vi "1.vi"() -> ()   [LabVIEW 2019]
uses:
  <vilib>/imath/engines/lvmath/Plug In/_Char/NIMS_CH_character datatype.ctl
  <vilib>/imath/engines/lvmath2/RunTimeEngine/Managers/WorkSpace/UID Generator.vi
  <vilib>/imath/engines/lvmath2/RunTimeEngine/BuiltInFunctions/close/NIMS_close(Enums).vi
  <vilib>/imath/engines/lvmath2/RunTimeEngine/RangeToken/NIMS_Range.vi
  <instcachedir>/0/NIMS_Range_FADF6ADDA3E145BB934C8BD4C7DAAB97.lvgen/NIMS_Range_FADF6ADDA3E145BB934C8BD4C7DAAB97_000.vi
  <vilib>/imathl/engines/lvmath/Functions/Error Handling/Create Error.vi
  <vilib>/imath/engines/lvmath/Plug In/_Char/NIMS_CH_Character RV to String.vi
  <vilib>/imath/engines/lvmath2/RunTimeEngine/BuiltInFunctions/random/NIMS_random.vi
  <vilib>/imath/engines/lvmath2/RunTimeEngine/IndexRead/NIMS M(S).vi
  <instcachedir>/0/NIMS M(S)_B826C018497E4940AE96BD27B540B6FB.lvgen/NIMS M(S)_B826C018497E4940AE96BD27B540B6FB_000.vi
  <vilib>/imath/engines/lvmath2/RunTimeEngine/ArithmeticOperatorToken/NIMS_ArithmeticOperator_plus.vi
  <instcachedir>/0/NIMS_ArithmeticOperator_plus_5C9385B0197D46E2B844C41E02F9EC39.lvgen/NIMS_ArithmeticOperator_plus_5C9385B0197D46E2B844C41E02F9EC39_004.vi
  <vilib>/imath/engines/lvmath2/RunTimeEngine/ErrorHandling/NIMS_Create Error From Enums.vi
  <vilib>/imath/engines/lvmath2/RunTimeEngine/BuiltInFunctions/randnormal/NIMS_randnormal(1,I32).vi
  <vilib>/imath/engines/lvmath2/RunTimeEngine/ErrorHandling/NIMS_Error From Error Code.vi
  <vilib>/imath/engines/lvmath/Functions/Error Handling/MergeErrorsWrapper.vi
  <vilib>/imath/engines/lvmath2/RunTimeEngine/BuiltInFunctions/fft/NIMS_fft(GV).vi
  <instcachedir>/0/NIMS_fft(GV)_4C6467FC22F84E4BA42517A07EF978B0.lvgen/NIMS_fft(GV)_4C6467FC22F84E4BA42517A07EF978B0_000.vi
  <vilib>/imath/engines/lvmath2/RunTimeEngine/BuiltInFunctions/abs/NIMS_abs(signed).vi
  <instcachedir>/0/NIMS_abs(signed)_C4FCB8E6058B49B797C7C8D53CA5F6EC.lvgen/NIMS_abs(signed)_C4FCB8E6058B49B797C7C8D53CA5F6EC_006.vi
  <vilib>/imath/engines/lvmath2/RunTimeSupport/NIMS_Error if Not Equal.vi
  <vilib>/imath/engines/lvmath2/RunTimeEngine/IndexRead/NIMS V(V).vi
  <instcachedir>/0/NIMS V(V)_298D9CB7BFEB42B8BC8D9C3C28AE8C70.lvgen/NIMS V(V)_298D9CB7BFEB42B8BC8D9C3C28AE8C70_000.vi
  <vilib>/imath/engines/lvmath2/RunTimeEngine/BuiltInFunctions/psd_periodogram/NIMS_psd_periodogram().vi
  <instcachedir>/0/NIMS_psd_periodogram()_F7AFC2F0C6104ABD8A95B4677FDE116B.lvgen/NIMS_psd_periodogram()_F7AFC2F0C6104ABD8A95B4677FDE116B_000.vi
  <vilib>/imath/engines/lvmath2/RunTimeEngine/Managers/SymbolTable/Clear UID.vi
  <vilib>/imath/engines/lvmath2/RunTimeEngine/NodeEndStatement/NIMS_NodeEndStatement_Output.vi
  <instcachedir>/0/NIMS_NodeEndStatement_Output_53EC0D466D134D7ABD903AC30B43404B.lvgen/NIMS_NodeEndStatement_Output_53EC0D466D134D7ABD903AC30B43404B_005.vi
  <instcachedir>/0/NIMS_NodeEndStatement_Output_53EC0D466D134D7ABD903AC30B43404B.lvgen/NIMS_NodeEndStatement_Output_53EC0D466D134D7ABD903AC30B43404B_000.vi
  <vilib>/imath/engines/lvmath2/RunTimeEngine/ErrorHandling/NIMS_Finalize Error.vi
  <vilib>/imath/engines/lvmath2/RunTimeEngine/Managers/SymbolTable/NIMS_WorkSpace.lvlib
panel:
  out "periodogram函数估计功率谱":cluster{"f":dbl[], "logsx2":dbl[]}(graph)
  out "周期图法估计功率谱":cluster{"f":dbl[], "logsx1":dbl[]}(graph)
  out "随机信号时域波形":dbl[](graph)
  in  "A2":dbl=5.0
  in  "A1":dbl=2.0
  in  "f2":dbl=100.0
  in  "f1":dbl=30.0
  in  "fs":dbl=1000.0
  in  "N":dbl=1024.0
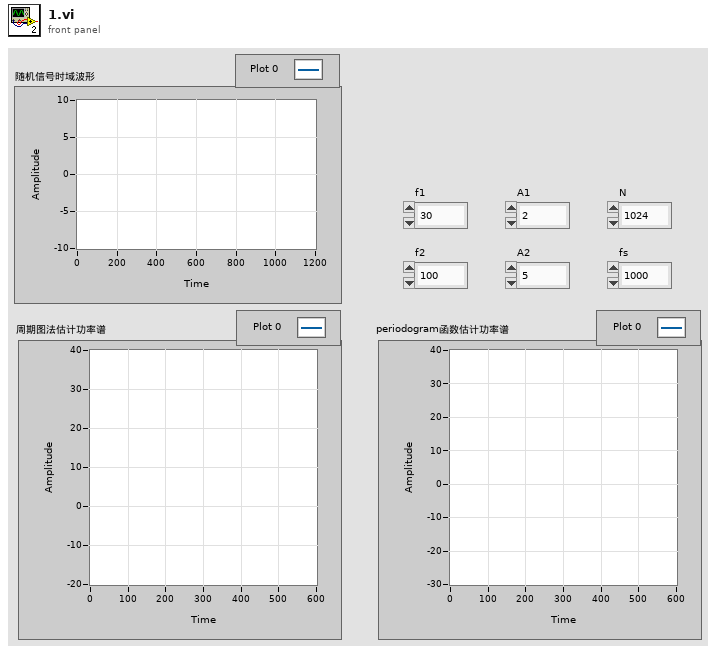
[diagram p1: front panel]
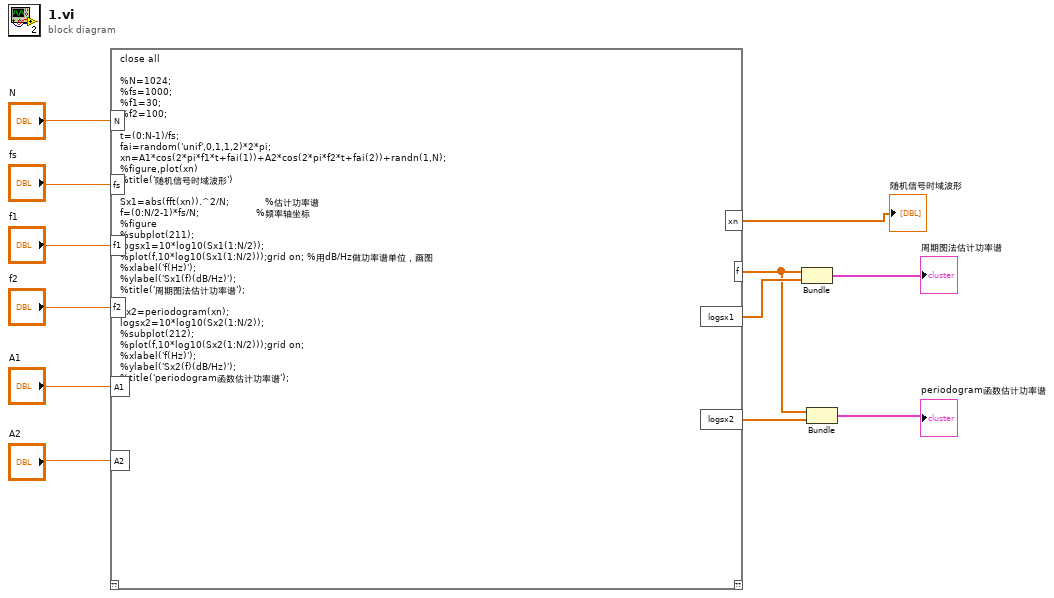
[diagram p0: block diagram]
diagram:
  n1 = mathscript code="close all\n\n%N=1024;\n%fs=1000;\n%f1=30;\n%f2=100;\n\nt=(0:N-1)/fs;\nfai=random('unif',0,1,1,2)*2*pi;\nxn=A1*cos(2*pi*f1*t+fai(1))+A2*cos(2*pi*f2*t+fai(2))+randn(1,N);\n%figure,plot(xn)\n%title('随机信号时域波形')\n\nSx1=abs(fft(xn)).^2/N;            %估计功率谱\nf=(0:N/2-1)*fs/N;                   %频率轴坐标\n%figure\n%subplot(211);\nlogsx1=10*log10(Sx1(1:N/2));\n%plot(f,10*log10(Sx1(1:N/2)));grid on; %用dB/Hz做功率谱单位，画图\n%xlabel('f(Hz)');\n%ylabel('Sx1(f)(dB/Hz)');\n%title('周期图法估计功率谱');\n\nSx2=periodogram(xn);\nlogsx2=10*log10(Sx2(1:N/2));\n%subplot(212);\n%plot(f,10*log10(Sx2(1:N/2)));grid on;\n%xlabel('f(Hz)');\n%ylabel('Sx2(f)(dB/Hz)');\n%title('periodogram函数估计功率谱');"("N"="N", "fs"="fs", "f1"="f1", "f2"="f2", "A1"="A1", "A2"="A2") -> ("xn"=→"随机信号时域波形":dbl[], "logsx1"=w6:cdb[], "logsx2"=w4:cdb[], "f"=w5:dbl[])  [unwired: 1 in, 1 out]
  n2 = Bundle("f"=w5, "logsx1"=w6) -> (→"周期图法估计功率谱":cluster{"f":dbl[], "logsx1":cdb[]})  [unwired: 1 in]
  n3 = Bundle("f"=w5, "logsx2"=w4) -> (→"periodogram函数估计功率谱":cluster{"f":dbl[], "logsx2":cdb[]})  [unwired: 1 in]
